vi "Get Nsamples ILD1420.vi"(0 "COM port":refnum<visa-resource-name>, 7 "N samples":i32=2000 min=0, 9 "Measuring range (mm)":u8(ring)=4 items=["10", "25", "50", "100", "200"], 11 "Auto laser off":bool=TRUE) -> (4 "d (mm)":dbl[](array[numeric]), 15 "Error out":errorcluster)   [LabVIEW 2016]
panel:
  out "Samples acquired":i32
  out "Distance":dbl(graph)
  out "Bits":bool[][](array[boolean])
  # "mm"
  # "PN 12/08/2016"
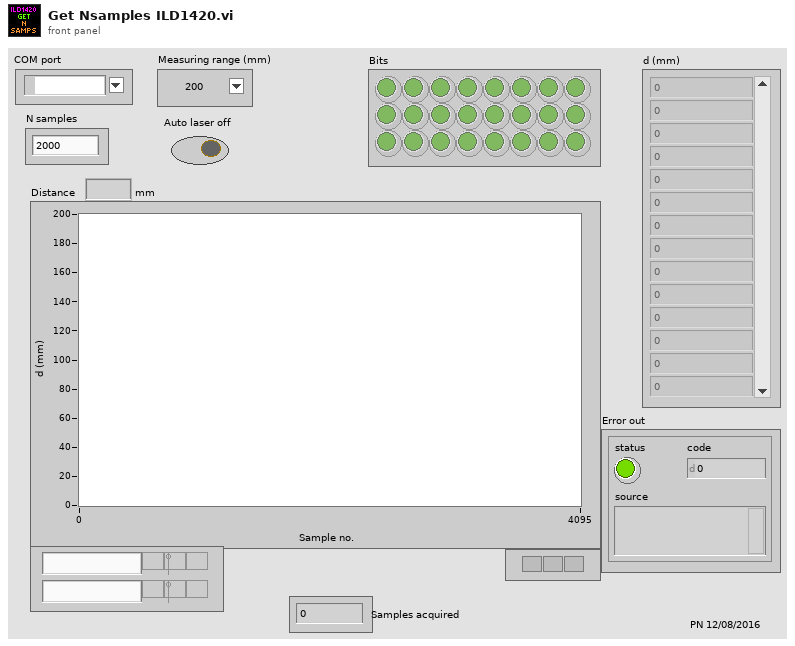
[diagram p1: front panel]
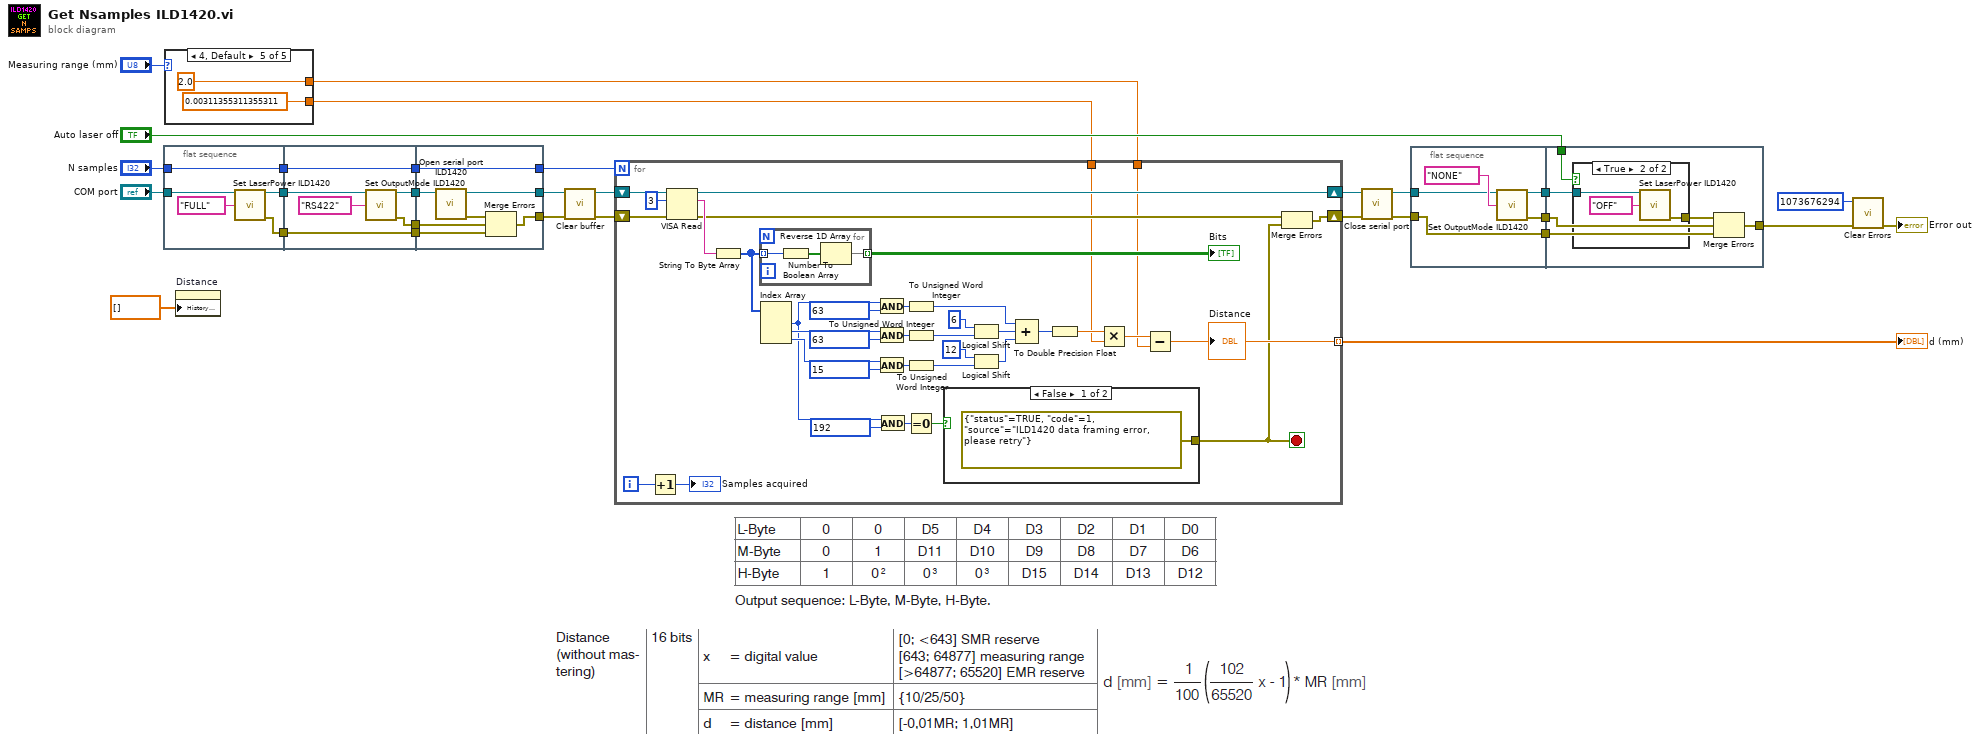
[diagram p0: block diagram]
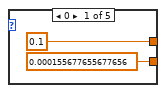
[diagram p2: hidden frame]
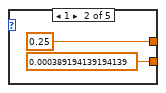
[diagram p3: hidden frame]
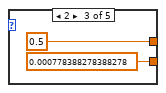
[diagram p4: hidden frame]
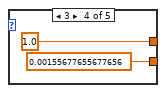
[diagram p5: hidden frame]
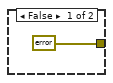
[diagram p6: hidden frame]
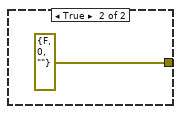
[diagram p7: hidden frame]
diagram:
  n1 = flat-sequence {
    tunnel: "N samples" -> [w33]
    tunnel: "COM port" -> [w32]
    tunnel: [w33] -> w19
    tunnel: [w32] -> w18
    tunnel: [w31] -> w16
    tunnel: [w37] -> w26
    tunnel: [w36] -> w25
    tunnel: [w35] -> w24
    tunnel: w19 -> [w35]
    tunnel: w18 -> [w37]
    tunnel: [w34] -> w17
    tunnel: w16 -> [w34]
    tunnel: [w45] -> w4
    tunnel: [w41] -> w2
    tunnel: w26 -> [w44]
    tunnel: w25 -> [w42]
    tunnel: w24 -> [w40]
    tunnel: [w40] -> w22
    tunnel: w17 -> [w39]
    frame #0 {
      n2 = call "Set LaserPower ILD1420.vi"("COM port"=w32, "Power"="FULL") -> ("Error out"=w31:errorcluster)  [unwired: 13 in]
    }
    frame #1 {
      n3 = call "Set OutputMode ILD1420.vi"("COM port"=w37, "Output mode"="RS422") -> ("Error out"=w36:errorcluster)  [unwired: 13 in]
    }
    frame #2 {
      n4 = call "Open serial port ILD1420.vi"("VISA resource name"=w44) -> ("Error out"=w43:errorcluster, "VISA resource name out"=w45:refnum<visa-resource-name>)  [unwired: 9 in]
      n5 = Merge Errors(w43, w42, w39) -> (w41:errorcluster)
    }
  }
  n6 = case shown="4, Default" "Measuring range (mm)" {
    tunnel: [0.1 0.25 0.5 1.0 2.0] -> w9
    tunnel: [0.000155677655677656 0.000389194139194139 0.000778388278388278 0.00155677655677656 0.00311355311355311] -> w8
    frame 0 {
    }
    frame 1 {
    }
    frame 2 {
    }
    frame 3 {
    }
    frame 4, Default {
    }
  }
  n7 = property on="Distance" class="WFChart (strict)"("History Data"=dbl[] []) -> ()  [unwired: 2 in, 2 out]
  n8 = call "Clear buffer.vi"("Error In"=w2, "VISA resource name"=w4) -> ("Error Out"=w1:errorcluster, "VISA resource name out"=w3:refnum<visa-resource-name>)  [unwired: 8 in]
  n9 = for {
    N: w22 -> [_]
    shift-right: [w92] -> w7
    shift-left: w3 -> [w88]
    shift-right: [w61] -> w6
    shift-left: w1 -> [w87]
    tunnel: [w67] -> w29 mode=indexing
    tunnel: w8 -> [w57]
    tunnel: w9 -> [w56]
    i -> [w59]
    stop <- w60 stop-if-true
    n10 = Increment(x=w59) -> (x+1=→"Samples acquired":i32)
    n11 = VISA Read(VISA resource name=w88, byte count=u32 3, error in (no error)=w87) -> (VISA resource name out=w92:refnum<visa-resource-name>, read buffer=w89:string, error out=w62:errorcluster)  [unwired: 1 out]
    n12 = String To Byte Array(string=w89) -> (unsigned byte array=w68:u8[])
    n13 = for {
      tunnel: w68 -> [w97] mode=indexing
      tunnel: [w95] -> w90 mode=indexing
      n14 = Number To Boolean Array(number=w97) -> (Boolean array=w96:bool[])
      n15 = Reverse 1D Array(array=w96) -> (reversed array=w95:bool[])
    }
    "Bits" <- w90
    n16 = Index Array(array=w68) -> (element #1=w65:u8, element #2=w73:u8, element #3=w75:u8)  [unwired: 3 in]
    n17 = And(x=w65, y=u8 63) -> (x .and. y?=w83:u8)
    n18 = And(x=w73, y=u8 63) -> (x .and. y?=w76:u8)
    n19 = And(x=w75, y=u8 15) -> (x .and. y?=w79:u8)
    n20 = And(x=w65, y=u8 192) -> (x .and. y?=w64:u8)
    n21 = To Unsigned Word Integer(number=w83) -> (unsigned 16bit integer=w84:u16)
    n22 = To Unsigned Word Integer(number=w76) -> (unsigned 16bit integer=w85:u16)
    n23 = To Unsigned Word Integer(number=w79) -> (unsigned 16bit integer=w86:u16)
    n24 = Equal To 0?(x=w64) -> (x = 0?=w63:bool)
    n25 = case shown="False" w63 {
      tunnel: [errorcluster {"status"=TRUE, "code"=1, "source"="ILD1420 data framing error, please retry"} ("error out") errorcluster {"status"=FALSE, "code"=0, "source"=""} ("error out")] -> w60
      frame False {
      }
      frame True {
      }
    }
    n26 = Logical Shift(y=i16 6, x=w85) -> (x << y=w82:u16)
    n27 = Logical Shift(y=i16 12, x=w86) -> (x << y=w81:u16)
    n28 = Compound Arithmetic op=ADD(w84, w82, w81) -> (w80:u16)
    n29 = To Double Precision Float(number=w80) -> (double precision float=w69:dbl)
    n30 = Multiply(x=w69, y=w57) -> (x*y=w70:dbl)
    n31 = Subtract(x=w70, y=w56) -> (x-y=w67:dbl)
    "Distance" <- w67
    n32 = Merge Errors(w62, w60) -> (w61:errorcluster)
  }
  "d (mm)" <- w29
  n33 = call "Close serial port.vi"("Error in"=w6, "VISA resource name"=w7) -> ("Error out"=w5:errorcluster)  [unwired: 9 in]
  n34 = flat-sequence {
    tunnel: w7 -> [w100]
    tunnel: w5 -> [w98]
    tunnel: [w100] -> w15
    tunnel: [w99] -> w14
    tunnel: [w98] -> w13
    tunnel: w15 -> [w107]
    tunnel: w14 -> [w105]
    tunnel: w13 -> [w104]
    tunnel: [w103] -> w12
    tunnel: "Auto laser off" -> [w102]
    frame #0 {
      n35 = call "Set OutputMode ILD1420.vi"("COM port"=w100, "Output mode"="NONE") -> ("Error out"=w99:errorcluster)  [unwired: 13 in]
    }
    frame #1 {
      n36 = case shown="True" w102 {
        tunnel: w107 -> [_ w110]
        tunnel: [errorcluster {"status"=FALSE, "code"=0, "source"=""} ("Error out") w109] -> w106
        frame False {
        }
        frame True {
          n37 = call "Set LaserPower ILD1420.vi"("COM port"=w110, "Power"="OFF") -> ("Error out"=w109:errorcluster)  [unwired: 13 in]
        }
      }
      n38 = Merge Errors(w106, w105, w104) -> (w103:errorcluster)
    }
  }
  n39 = call <vilib>:"Clear Errors.vi"("error in (no error)"=w12, "specific error code to clear (0: all)"=1073676294) -> ("error out"=→"Error out":errorcluster)  [unwired: 4 in, 1 out]
